vi "main pop-up.vi"(8 "error in":errorcluster, 11 "Pop-up Input":T2) -> (0 "error out":errorcluster, 3 "Pop-up Output":T1)   [LabVIEW 2019, in "ZenGage v3.0 UI.lvclass"]
uses:
  ZenGage v3.0 UI.lvclass
  Controls/Pop-up Output.ctl
  Common/Controls/Pop-up Input.ctl
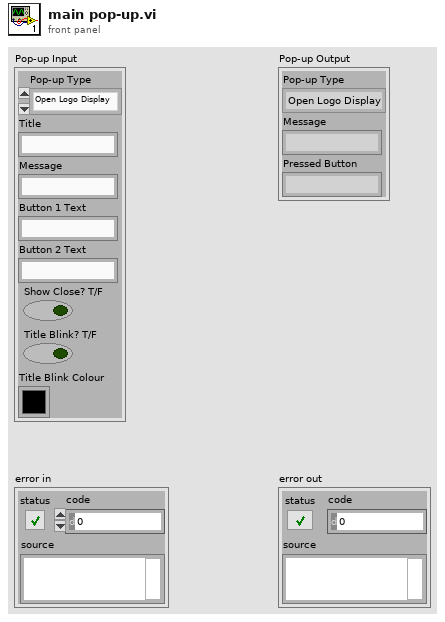
[diagram p1: front panel]
types:
  T1 = typedef "ZenGage v3.0 UI.lvclass/Pop-up Output.ctl" = cluster{"Pop-up Type":enum16{"Open Logo Display", "Close Logo Display", "Open Loading Bar", "Close Loading Bar", "Open Alert Display", "Close Alert Display", "One button dialog box", "Two button dialog box", "User Authentication"}, "Message":string, "Pressed Button":string}
  T2 = typedef "Pop-up Input.ctl" = cluster{"Pop-up Type":enum16{"Open Logo Display", "Close Logo Display", "Open Loading Bar", "Close Loading Bar", "Open Alert Display", "Close Alert Display", "One button dialog box", "Two button dialog box", "User Authentication"}, "Title":string, "Message":string, "Button 1 Text":string, "Button 2 Text":string, "Show Close? T/F":bool, "Title Blink? T/F":bool, "Title Blink Colour":u32}
  T3 = enum16{"Open Logo Display", "Close Logo Display", "Open Loading Bar", "Close Loading Bar", "Open Alert Display", "Close Alert Display", "One button dialog box", "Two button dialog box", "User Authentication"}
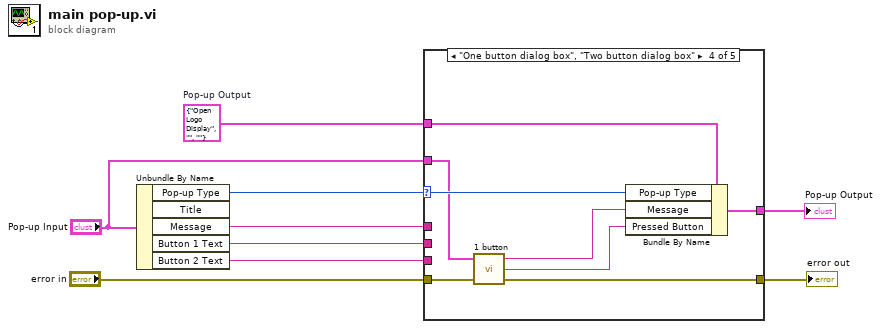
[diagram p0: block diagram]
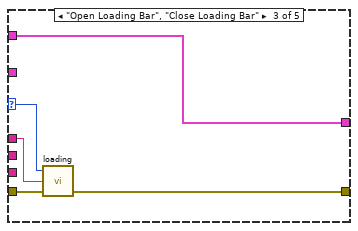
[diagram p4: hidden frame]
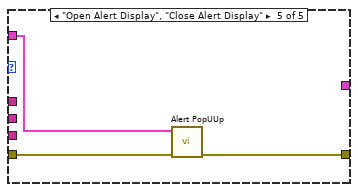
[diagram p5: hidden frame]
diagram:
  w3 = T1 {"Pop-up Type"=enum."Open Logo Display", "Message"="", "Pressed Button"=""}  # Pop-up Output
  n1 = Unbundle By Name("Pop-up Input") -> ("Pop-up Type"=w7:T3, "Message"=w6:string, "Button 1 Text"=w5:string, "Button 2 Text"=w4:string)  [unwired: 1 out]
  n2 = case shown="\"One button dialog box\", \"Two button dialog box\"" w7 {
    selector: w7 -> [_ _ w14 w22 _]
    tunnel: w6 -> [_ _ w18 _ _]
    tunnel: w5 -> [_ _ _ _ _]
    tunnel: "error in" -> [w11 w12 w17 w26 w29]
    tunnel: [w11 w12 w16 w25 w27] -> w9
    tunnel: w4 -> [_ _ _ _ _]
    tunnel: w3 -> [w10 w13 w15 w21 _]
    tunnel: [w10 w13 w15 w20 _] -> w2
    tunnel: "Pop-up Input" -> [_ _ _ w19 w28]
    frame Default {
    }
    frame "Open Logo Display", "Close Logo Display" {
      # "Zentron Logo is displayed"
    }
    frame "Open Loading Bar", "Close Loading Bar" {
      n3 = call "loading.vi"("error in"=w17, "Message"=w18, "Pop-up Type"=w14) -> ("error out"=w16:errorcluster)  [unwired: 2 in]
    }
    frame "One button dialog box", "Two button dialog box" {
      n4 = call "1 button.vi"("error in"=w26, "Pop-up Input"=w19) -> ("error out"=w25:errorcluster, "Pressed Button"=w24:string, "Message"=w23:string)  [unwired: 1 in]
      n5 = Bundle By Name(cluster=w21, "Pop-up Type"=w22, "Message"=w23, "Pressed Button"=w24) -> (w20:T1)
    }
    frame "Open Alert Display", "Close Alert Display" {
      n6 = call "Alert PopUUp.vi"("error in (no error)"=w29, "Pop-up Input"=w28) -> ("error out"=w27:errorcluster)  [unwired: 9 in]
    }
  }
  "error out" <- w9
  "Pop-up Output" <- w2
